vi "LVUSBRH2_VISA_CMD_led_onoff.vi"(8 "error in (no error)":errorcluster caption="error in(no errro)", 9 "Sw":bool, 10 "CH#(1)":i32=1, 11 "VISA rssc":refnum<visa-resource-name>) -> (0 "error out":errorcluster, 3 "VISA rssc out":refnum<visa-resource-name>)   [LabVIEW 2020]
panel:
  out "rcv string":string
  out "cmd string":string
  # "LED1=赤\nLED2=緑"
  # "Response:\nLED[12]=ON|OFF\\r\\n"
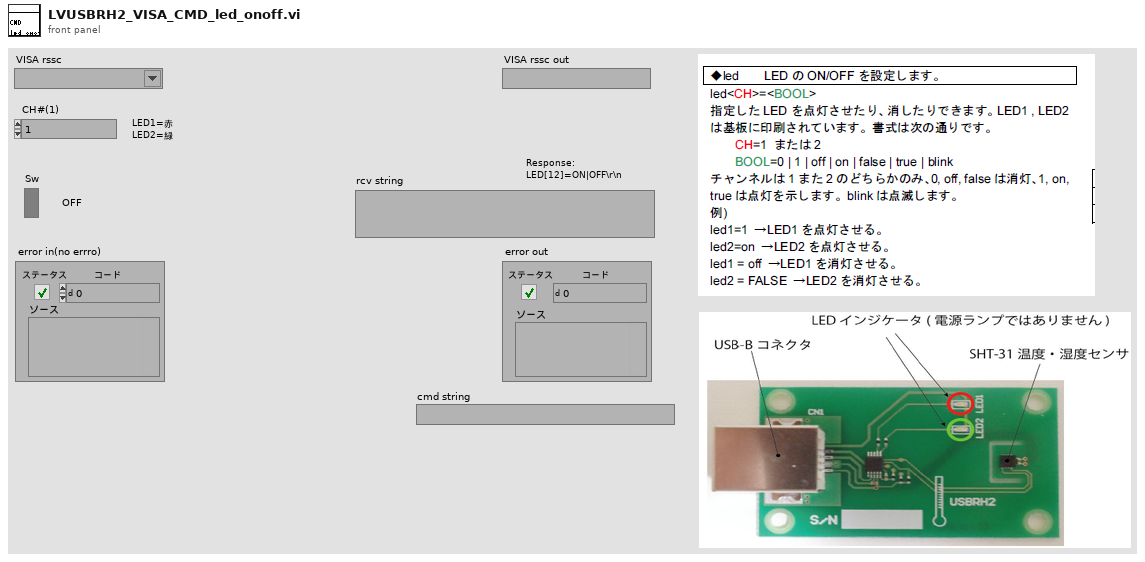
[diagram p1: front panel]
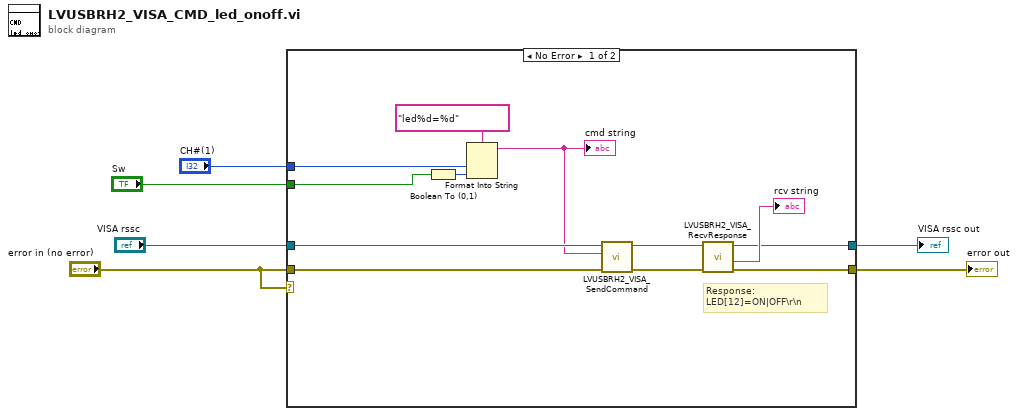
[diagram p0: block diagram]
diagram:
  n1 = case shown="No Error" "error in (no error)" {
    tunnel: "VISA rssc" -> [w18 w20]
    tunnel: [w7 w20] -> w5
    tunnel: "error in (no error)" -> [w17 w19]
    tunnel: [w8 w19] -> w4
    tunnel: "Sw" -> [w13 _]
    tunnel: "CH#(1)" -> [w14 _]
    frame No Error {
      # "Response:\nLED[12]=ON|OFF\\r\\n"
      n2 = Boolean To (0,1)(Boolean=w13) -> (0, 1=w12:i16)
      n3 = Format Into String(format string="led%d=%d" ("形式文字列"), w14, w12) -> (resulting string=w15:string)  [unwired: 2 in, 1 out]
      "cmd string" <- w15
      n4 = call "LVUSBRH2_VISA_SendCommand.vi"("error in (no error)"=w17, "cmd string"=w15, "VISA rssc"=w18) -> ("error out"=w9:errorcluster, "VISA rssc out"=w10:refnum<visa-resource-name>)  [unwired: 7 in]
      n5 = call "LVUSBRH2_VISA_RecvResponse.vi"("error in (no error)"=w9, "VISA rssc"=w10) -> ("error out"=w8:errorcluster, "rcv string"=→"rcv string":string, "VISA rssc out"=w7:refnum<visa-resource-name>)  [unwired: 7 in]
    }
    frame Error {
    }
  }
  "VISA rssc out" <- w5
  "error out" <- w4
